vi "ISX3_Cmd_SetSyncTimevi.vi"() -> ()   [LabVIEW 2012, in "Sciospec ISX3 Impedance Analyzer.lvlib"]
uses:
  Sciospec ISX3 Impedance Analyzer.lvlib
panel:
  in  "Sync Time in µs":u32
  out "Set Sync Time Command":u8[](array[numeric])
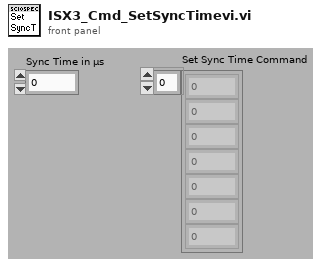
[diagram p1: front panel]
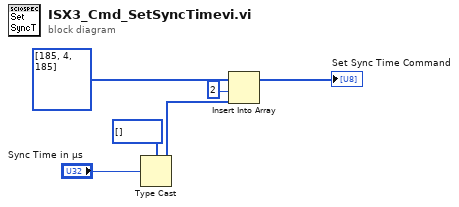
[diagram p0: block diagram]
diagram:
  n1 = Type Cast(type=u8[] [], x="Sync Time in µs") -> (*(type *) &x=w3:u8[])
  n2 = Insert Into Array(array=u8[] [185, 4, 185], index=2 ("Index"), new element=w3) -> (→"Set Sync Time Command":u8[])
